vi "programal 1 tercer parcial.vi"() -> ()   [LabVIEW 2011]
uses:
  control 1 tercer parcial.ctl
panel:
  out "Array":T1(array[cluster]) {"temperatura3" scale=0.0..60.0; "temperatura2" scale=0.0..60.0; "Temperatura" scale=0.0..60.0}
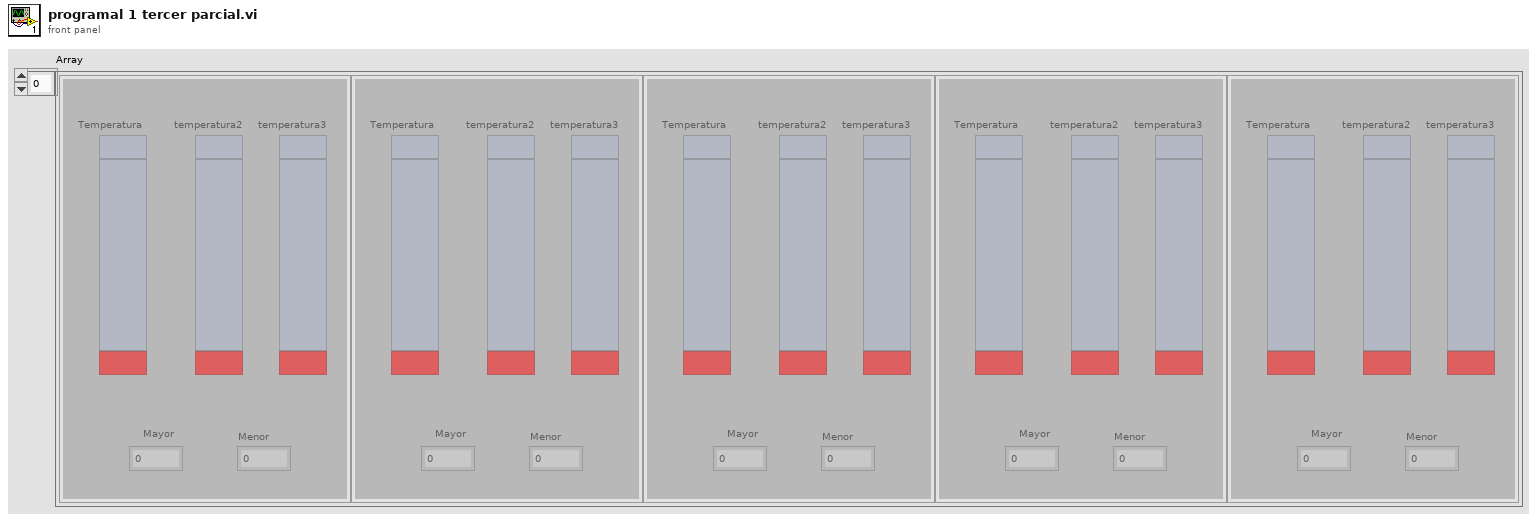
[diagram p1: front panel]
types:
  T1 = cluster{"Temperatura":i32, "temperatura2":i32, "temperatura3":i32, "Mayor":dbl, "Menor":dbl}[]
  T2 = typedef "control 1 tercer parcial.ctl" = enum16{"iniciar arreglo", "Ingresar temperatura", "Obtener maximo y minimo", "finalizar"}
  T3 = cluster{"Temperatura":i32, "temperatura2":i32, "temperatura3":i32, "Mayor":dbl, "Menor":dbl}
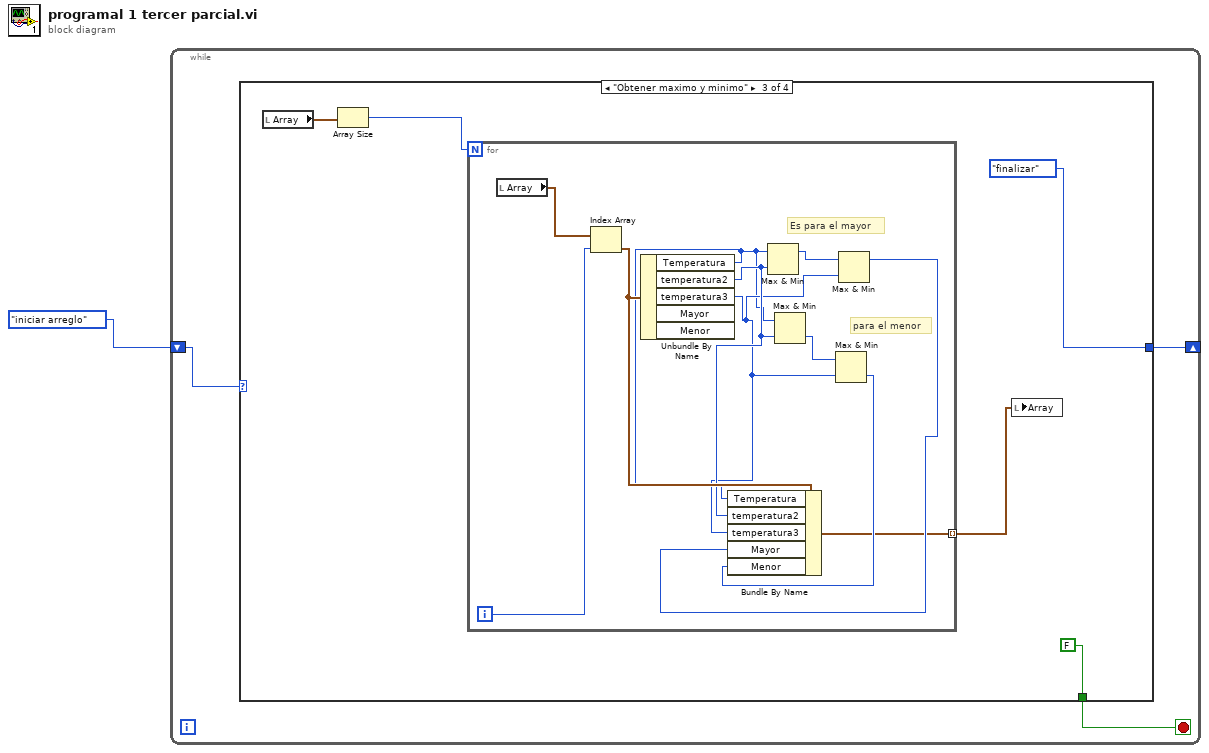
[diagram p0: block diagram]
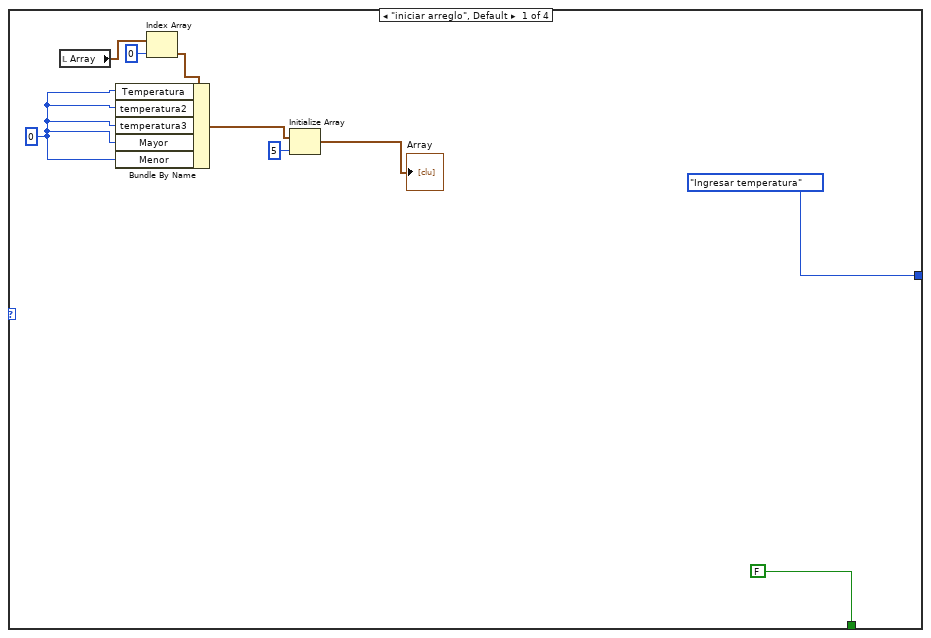
[diagram p2: hidden frame]
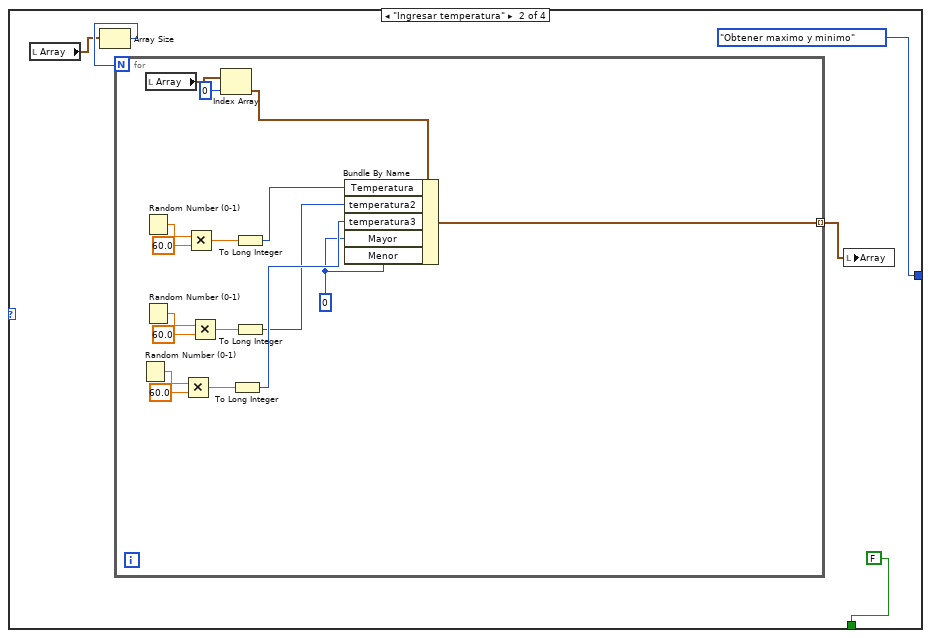
[diagram p3: hidden frame]
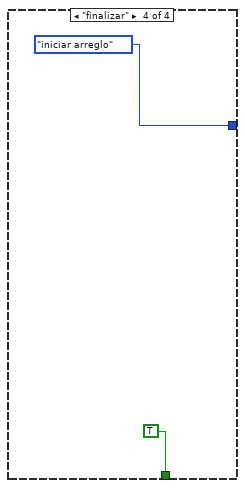
[diagram p4: hidden frame]
diagram:
  n1 = while {
    shift-right: [w3] -> _
    shift-left: control_1_tercer_parcial."iniciar arreglo" -> [w4]
    stop <- w2 stop-if-true
    n2 = case shown="\"Obtener maximo y minimo\"" w4 {
      tunnel: [control_1_tercer_parcial."Ingresar temperatura" control_1_tercer_parcial."Obtener maximo y minimo" control_1_tercer_parcial."finalizar" control_1_tercer_parcial."iniciar arreglo"] -> w3
      tunnel: [FALSE FALSE FALSE TRUE] -> w2
      frame "iniciar arreglo", Default {
        w8 = 0
        n3 = local read "Array"() -> (w11:T1)
        n4 = Index Array(array=w11, index=0) -> (element=w9:T3)
        n5 = Bundle By Name(cluster=w9, "Temperatura"=w8, "temperatura2"=w8, "temperatura3"=w8, "Mayor"=w8, "Menor"=w8) -> (w12:T3)
        n6 = Initialize Array(w12, 5 ("dimension size")) -> (→"Array":T1)
      }
      frame "Ingresar temperatura" {
        n7 = local read "Array"() -> (w17:T1)
        n8 = Array Size(array=w17) -> (size(s)=w18:i32)
        n9 = for {
          N: w18 -> [_]
          tunnel: [w20] -> w16 mode=indexing
          w19 = 0
          n10 = Random Number (0-1)() -> (number: 0 to 1=w25:dbl)
          n11 = Random Number (0-1)() -> (number: 0 to 1=w32:dbl)
          n12 = Random Number (0-1)() -> (number: 0 to 1=w26:dbl)
          n13 = local read "Array"() -> (w35:T1)
          n14 = Multiply(x=w25, y=60.0) -> (x*y=w23:dbl)
          n15 = Multiply(x=w32, y=60.0) -> (x*y=w30:dbl)
          n16 = Multiply(x=w26, y=60.0) -> (x*y=w28:dbl)
          n17 = Index Array(array=w35, index=0) -> (element=w33:T3)
          n18 = To Long Integer(number=w23) -> (32bit integer=w22:i32)
          n19 = To Long Integer(number=w30) -> (32bit integer=w29:i32)
          n20 = To Long Integer(number=w28) -> (32bit integer=w21:i32)
          n21 = Bundle By Name(cluster=w33, "Temperatura"=w29, "temperatura2"=w21, "temperatura3"=w22, "Mayor"=w19, "Menor"=w19) -> (w20:T3)
        }
        n22 = local write "Array"(w16) -> ()
      }
      frame "Obtener maximo y minimo" {
        n23 = local read "Array"() -> (w40:T1)
        n24 = Array Size(array=w40) -> (size(s)=w39:i32)
        n25 = for {
          N: w39 -> [_]
          tunnel: [w42] -> w38 mode=indexing
          i -> [w50]
          # "para el menor"
          # "Es para el mayor"
          n26 = local read "Array"() -> (w51:T1)
          n27 = Index Array(array=w51, index=w50) -> (element=w47:T3)
          n28 = Unbundle By Name(w47) -> ("Temperatura"=w41:i32, "temperatura2"=w46:i32, "temperatura3"=w45:i32)  [unwired: 2 out]
          n29 = Max & Min(x=w41, y=w46) -> (max(x,y)=w49:i32)  [unwired: 1 out]
          n30 = Max & Min(x=w41, y=w46) -> (min(x,y)=w48:i32)  [unwired: 1 out]
          n31 = Max & Min(x=w48, y=w45) -> (min(x,y)=w43:i32)  [unwired: 1 out]
          n32 = Max & Min(x=w49, y=w45) -> (max(x,y)=w44:i32)  [unwired: 1 out]
          n33 = Bundle By Name(cluster=w47, "Temperatura"=w41, "temperatura2"=w46, "temperatura3"=w45, "Mayor"=w44, "Menor"=w43) -> (w42:T3)
        }
        n34 = local write "Array"(w38) -> ()
      }
      frame "finalizar" {
      }
    }
  }
